vi "CPP-5168-TubingCompOnly.vi"() -> (5 "Plug in titles":string[](array[string]), 7 "Plug in values":string[](array[string]))   [LabVIEW 2015]
uses:
  Globals/Meas_global.vi
panel:
  in  "TubingCorrectionFile":path=path "/CentralDataCache/Preferences/Rig_Setups/All_Rigs/TubingCompensation/TUBECORR.20000.XLS"
  in  "inH20/V":dbl=1.0 caption="Calibration factor inH20/V"
  in  "Last non-pressure channel":string="Gen (Quiet)"
  out "Zeroes?":bool
  out "Zeroes":dbl[](array[numeric])
  out "Data":dbl[][](array[numeric]) caption="ZeroedCompensatedCalibratedData" format="%#_3g"
  out "ChannelNames":string[](array[string])
  # "Jan 2013: \"SurfaceCp\": 1.42857\"/V (x4V = 5.712\" total ?? -not a valid value??)(Need to confirm same or different TT than HFandPressure)\nJan 2013 \"HFandPressure\" 2.4377\"/V (x4V = 9.75\" Total: 1024or 768 table)(Forensics (Serial Error Logs) suggests TT#7, the 768MPS3 table, was used.)\nFeb 2012 \"PressureAnalysis\": 0.241\"/V (x4V = ~1\" total: 256 table)"
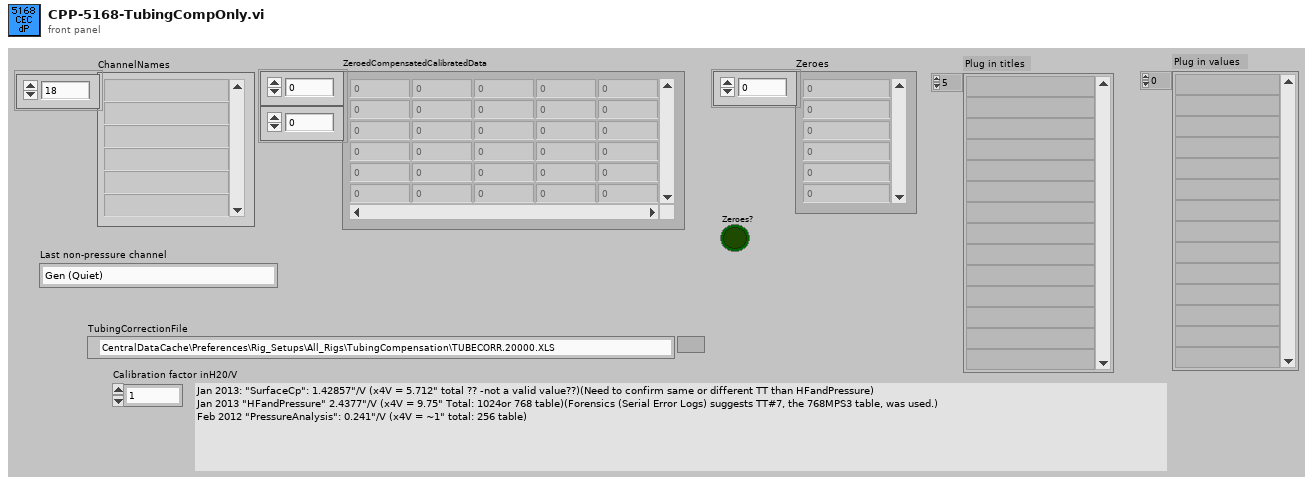
[diagram p1: front panel]
types:
  T1 = typedef "Analysis_info_cluster.ctl" = cluster{"Colour":u32, "Inst type":T2, "Inst name":string, "Symbol":string, "Code name":string, "Extra Info":string, "Inst Array":T3, "Extra Titles":string[], "Extra Values":string[], "U":dbl, "u^2":dbl, "u^3":dbl, "u^4":dbl, "Skew_u":dbl, "Kurt_u":dbl, "Sd Error in Mean":dbl, "% u'/U":dbl, "X":dbl, "Y":dbl, "Z":dbl, "Timescale integral to 25%":dbl, "Sd Error in Variance":dbl, "Calib File":path, "Calib Constants":dbl[], "Output Position":bool, "Full Stats":bool, "Av Sampling Rate":dbl, "Av No of Samples":dbl, "Total Meas Time (s)":dbl, "ADAM Ch Name":string}
  T2 = typedef "Inst_type.ctl" = enum16{"Propeller anemometer", "Raw voltage", "Pressure Transducer", "Pitot-static tube", "Preston tube", "Hot wire", "Cross wire 1", "Cross wire 2", "Generic Linear", "Generic Polynomial", "Generic BackPoly", "Fast FID", "Thermocouple", "Cold wire", "Pulsed Wire", "LDA Vel", "LDA Tran time", "LDA Arr time", "Microphone"}
  T3 = typedef "Instrument_Array.ctl" = enum16{"PWA", "LDA", "Analogue"}
  T4 = typedef "Time_Trace_Cluster.ctl" = cluster{"Weighting":dbl[], "Time (s)":dbl[], "Voltage":dbl[], "Eng Values":dbl[]}
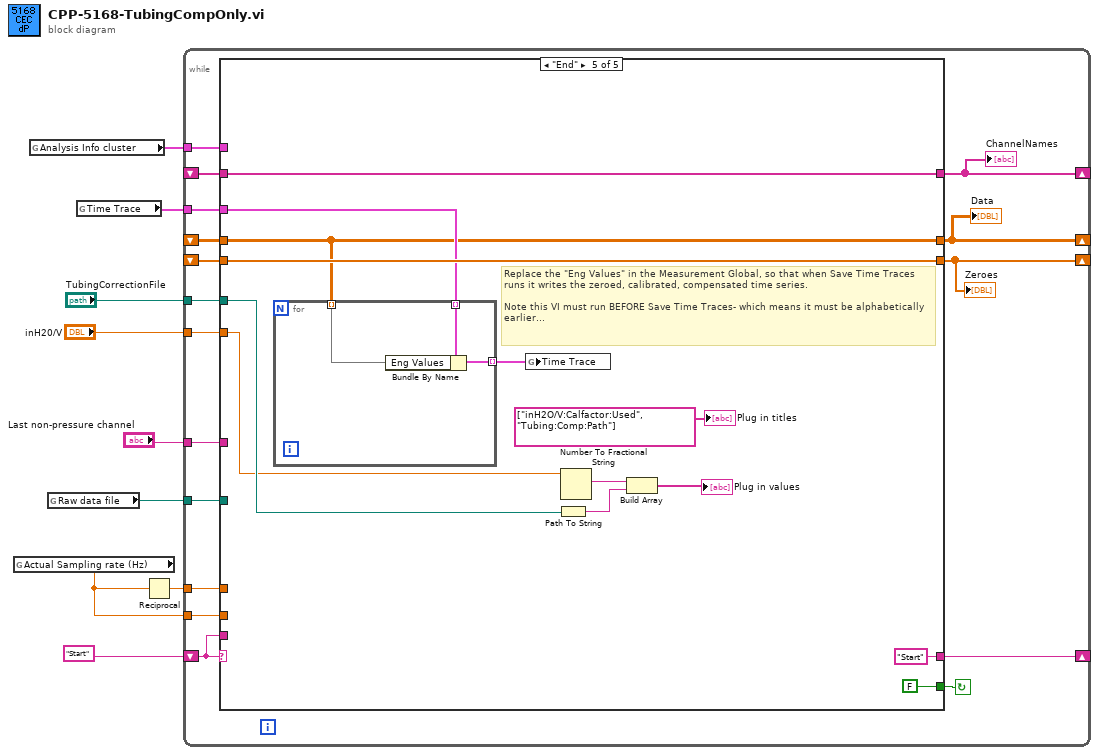
[diagram p0: block diagram]
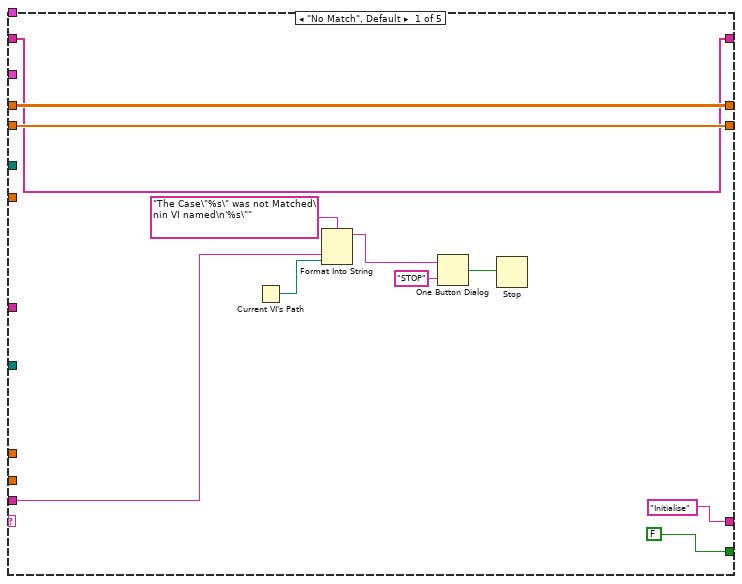
[diagram p2: hidden frame]
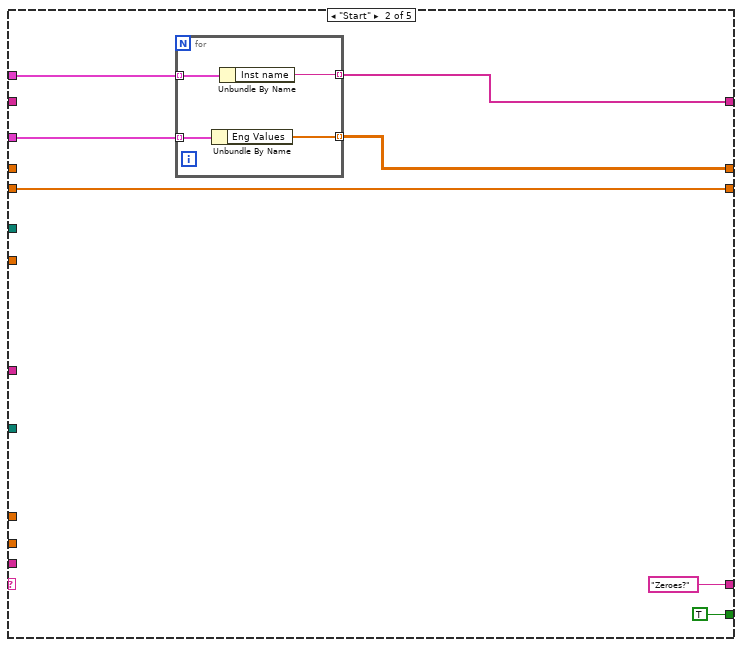
[diagram p3: hidden frame]
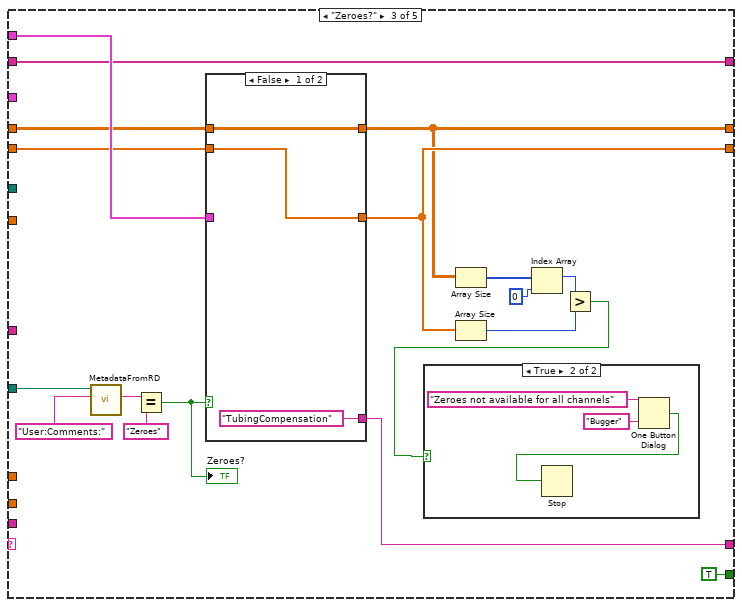
[diagram p4: hidden frame]
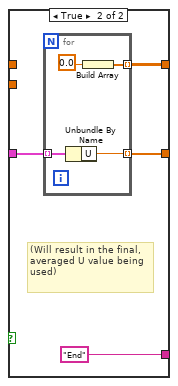
[diagram p6: hidden frame]
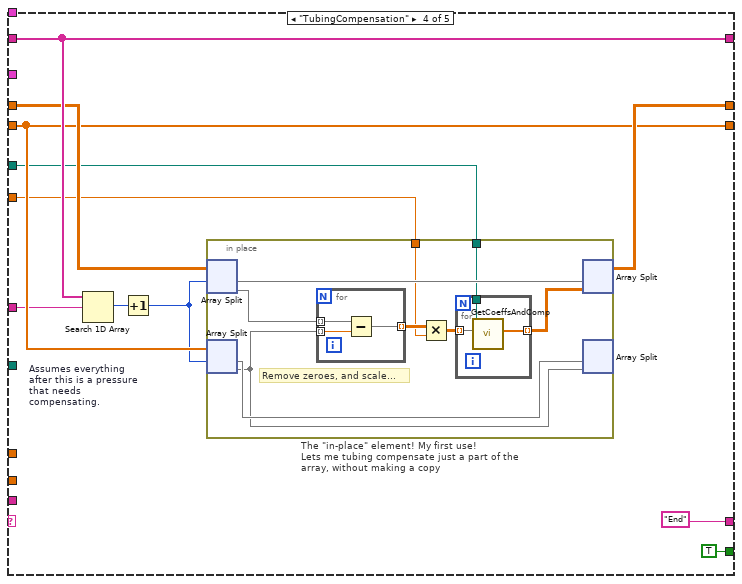
[diagram p7: hidden frame]
diagram:
  n1 = global read "Meas_global.vi" "Actual Sampling rate (Hz)"() -> (w8:dbl)
  n2 = global read "Meas_global.vi" "Analysis Info cluster"() -> (w5:T1[])
  n3 = global read "Meas_global.vi" "Raw data file"() -> (w6:path)
  n4 = global read "Meas_global.vi" "Time Trace"() -> (w4:T4[])
  n5 = Reciprocal(x=w8) -> (1/x=w7:dbl)
  n6 = while {
    shift-left: "Start" -> [w24]
    shift-right: [w25] -> _
    tunnel: w8 -> [w23]
    tunnel: w7 -> [w22]
    tunnel: w6 -> [w19]
    shift-right: [w18] -> _
    shift-left: _ -> [w17]
    shift-right: [w16] -> _
    shift-left: _ -> [w21]
    tunnel: w5 -> [w15]
    tunnel: w4 -> [w14]
    shift-right: [w13] -> _
    shift-left: _ -> [w20]
    tunnel: "TubingCorrectionFile" -> [w12]
    tunnel: "inH20/V" -> [w11]
    tunnel: "Last non-pressure channel" -> [w10]
    stop <- w26 continue-if-true
    n7 = case shown="\"End\"" w24 {
      tunnel: [FALSE TRUE ("Processing last block?") TRUE ("Processing last block?") TRUE ("Processing last block?") FALSE ("Processing last block?")] -> w26
      tunnel: ["Initialise" "Zeroes?" w60 "End" ("f") "Start" ("f")] -> w25
      tunnel: w24 -> [w32 _ _ _ _]
      tunnel: w23 -> [_ _ _ _ _]
      tunnel: w22 -> [_ _ _ _ _]
      tunnel: w21 -> [w28 _ w49 w86 w114]
      tunnel: w20 -> [w27 _ w51 w88 w107]
      tunnel: w19 -> [_ _ w66 _ _]
      tunnel: [w29 w42 w59 w85 w117] -> w18
      tunnel: w17 -> [w29 w42 w52 w85 w117]
      tunnel: [w28 w40 w50 w87 w114] -> w16
      tunnel: w15 -> [_ w39 w53 _ _]
      tunnel: w14 -> [_ w41 _ _ w116]
      tunnel: [w27 w38 w51 w88 w107] -> w13
      tunnel: w12 -> [_ _ _ w83 w112]
      tunnel: w11 -> [_ _ _ w82 w111]
      tunnel: w10 -> [_ _ _ w81 _]
      frame "No Match", Default {
        n8 = Current VI's Path() -> (path=w31:path)
        n9 = Format Into String(format string="The Case\"%s\" was not Matched\nin VI named\n'%s\"" ("Format String"), w32, w31) -> (resulting string=w35:string)  [unwired: 2 in, 1 out]
        n10 = One Button Dialog(message=w35, button name ("OK")="STOP") -> (true=w33:bool)
        n11 = Stop(stop? (T)=w33) -> ()
      }
      frame "Start" {
        n12 = for {
          tunnel: [w47] -> w40 mode=indexing
          tunnel: w41 -> [w48] mode=indexing
          tunnel: w39 -> [w46] mode=indexing
          tunnel: [w45] -> w38 mode=indexing
          n13 = Unbundle By Name(w48) -> ("Eng Values"=w47:dbl[])
          n14 = Unbundle By Name(w46) -> ("Inst name"=w45:string)
        }
      }
      frame "Zeroes?" {
        n15 = call "MetadataFromRD.vi"("ChannelName"="User:Comments:", "Raw data file"=w66) -> ("ValueString"=w63:string)  [unwired: 8 in, 1 out]
        n16 = Equal?(x=w63, y="Zeroes") -> (x = y?=w61:bool)
        "Zeroes?" <- w61
        n17 = case shown="False" w61 {
          tunnel: ["TubingCompensation" ("f") "End" ("f")] -> w60
          tunnel: [w71 w74] -> w59
          tunnel: w53 -> [_ w75]
          tunnel: w52 -> [w71 _]
          tunnel: [w70 w73] -> w50
          tunnel: w49 -> [w70 _]
          frame False {
          }
          frame True {
            # "(Will result in the final, averaged U value being used)"
            n18 = for {
              tunnel: w75 -> [w80] mode=indexing
              tunnel: [w79] -> w74 mode=indexing
              tunnel: [w77] -> w73 mode=indexing
              n19 = Unbundle By Name(w80) -> ("U"=w79:dbl)
              n20 = Build Array(0.0) -> (w77:dbl[])
            }
          }
        }
        n21 = Array Size(array=w50) -> (size(s)=w58:i32[])
        n22 = Array Size(array=w59) -> (size(s)=w57:i32)
        n23 = Index Array(array=w58, index=0) -> (element=w56:i32)
        n24 = Greater?(x=w56, y=w57) -> (0:w54:bool)
        n25 = case shown="True" w54 {
          frame False {
          }
          frame True {
            n26 = One Button Dialog(message="Zeroes not available for all channels", button name ("OK")="Bugger") -> (true=w67:bool)
            n27 = Stop(stop? (T)=w67) -> ()
          }
        }
      }
      frame "TubingCompensation" {
        n28 = Search 1D Array "Assumes everything after this is a pressure that needs compensating."(1D array=w88, element=w81) -> (index of element=w89:i32)  [unwired: 1 in]
        n29 = Increment(x=w89) -> (x+1=w84:i32)
        n30 = in-place "The \"in-place\" element! My first use!\nLets me tubing compensate just a part of the array, without making a copy" {
          in-place-border: w83 -> [w93]
          in-place-border: w82 -> [w92]
          # "Remove zeroes, and scale..."
          n31 = in-place-split #1(w86, w84) -> (w100:dbl[][], w97:dbl[][])
          n32 = in-place-split #2(w85, w84) -> (w95:dbl[], w94:dbl[])
          n33 = for {
            tunnel: [w103] -> w96 mode=indexing
            tunnel: w97 -> [w102] mode=indexing
            tunnel: w94 -> [w101] mode=indexing
            n34 = Subtract(x=w102, y=w101) -> (x-y=w103:dbl[])
          }
          n35 = Multiply(x=w96, y=w92) -> (x*y=w98:dbl[][])
          n36 = for {
            tunnel: w98 -> [w106] mode=indexing
            tunnel: [w105] -> w99 mode=indexing
            tunnel: w93 -> [w104]
            n37 = call "GetCoeffsAndComp.vi"("mutedData"=w106, "TubingCorrectionFile"=w104) -> ("boostedData"=w105:dbl[])  [unwired: 9 in]
          }
          n38 = in-place-split #1(w100, w99) -> (w87:dbl[][])  [unwired: 1 out]
          n39 = in-place-split #2(w95, w94) -> ()  [unwired: 2 out]
        }
      }
      frame "End" {
        # "Replace the \"Eng Values\" in the Measurement Global, so that when Save Time Traces runs it writes the zeroed, calibrated, compensated time series.\n\nNote this VI must run BEFORE Save Time Traces- which means it must be alphabetically earlier..."
        n40 = for {
          tunnel: w116 -> [w122] mode=indexing
          tunnel: [w121] -> w115 mode=indexing
          tunnel: w114 -> [w120] mode=indexing
          n41 = Bundle By Name(cluster=w122, "Eng Values"=w120) -> (w121:T4)
        }
        n42 = global write "Meas_global.vi" "Time Trace"(w115) -> ()
        n43 = Path To String(path=w112) -> (string=w109:string)
        n44 = Number To Fractional String(number=w111) -> (F-format string=w110:string)  [unwired: 3 in]
        n45 = Build Array(w110, w109) -> (→"Plug in values":string[])
        "Plug in titles" <- string[] ["inH2O/V:Calfactor:Used", "Tubing:Comp:Path"] ("Plug in titles")
      }
    }
    "Data" <- w16
    "Zeroes" <- w18
    "ChannelNames" <- w13
  }
